vi "range.vi"(9 "2D Pict origin":cluster{"x":dbl, "y":dbl}={"x"=200.0, "y"=200.0}, 10 "L 1":dbl=80.0, 11 "L 2":dbl=80.0) -> (3 "range picture":picture)   [LabVIEW 2024]
panel:
  out "end effector":cluster{dbl, dbl}={159.01647214211073, 1.9100783062530127} {"?" format="%.1f"; "?" format="%#.1f"}
  # "mm"
  # "mm"
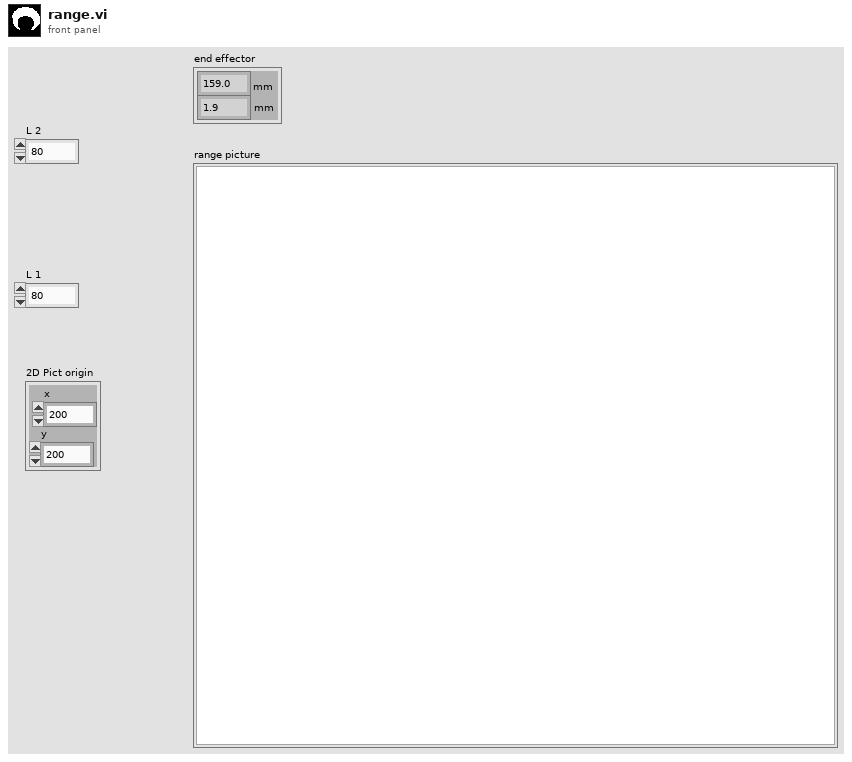
[diagram p1: front panel]
types:
  T1 = cluster{"Width":u16, "Style":enum32{"Solid", "Dash", "Dot", "DashDot", "DashDotDot"}}
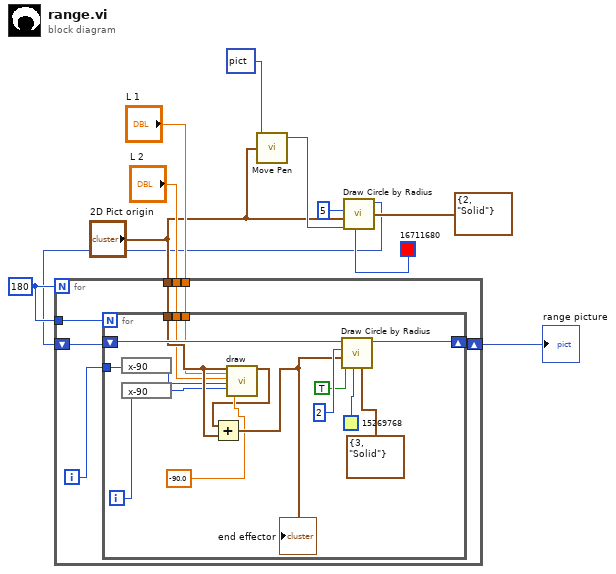
[diagram p0: block diagram]
diagram:
  w7 = 180
  n1 = call <vilib>:"Move Pen.vi"("new position"="2D Pict origin", "picture"=picture data[5B]) -> ("new picture"=w4:picture)  [unwired: 3 in]
  n2 = call <vilib>:"Draw Circle by Radius.vi"("pen"=T1 {"Width"=2, "Style"=enum."Solid"}, "color(black)"=u32 16711680, "pixel center"="2D Pict origin", "radius"=i16 5, "picture"=w4) -> ("new picture"=w1:picture)  [unwired: 6 in]
  n3 = for {
    N: w7 -> [_]
    tunnel: w7 -> [w18]
    shift-right: [w16] -> w6
    shift-left: w1 -> [w17]
    tunnel: "L 1" -> [w14]
    tunnel: "L 2" -> [w13]
    tunnel: "2D Pict origin" -> [w12]
    i -> [w15]
    n4 = for {
      N: w18 -> [_]
      shift-right: [w27] -> w16
      shift-left: w17 -> [w32]
      tunnel: w15 -> [w33]
      tunnel: w14 -> [w24]
      tunnel: w13 -> [w23]
      tunnel: w12 -> [w25]
      i -> [w34]
      n5 = expression code="x-90"(w33) -> (w22:i32)
      n6 = expression code="x-90"(w34) -> (w21:i32)
      n7 = call "draw.vi"("new position"=w25, "L 1"=w24, "L 2"=w23, "Angle1"=w22, "Angle 2"=w21, "bias"=-90.0) -> ("end effector"=w19:cluster{dbl, dbl})  [unwired: 9 in, 4 out]
      n8 = Add(x=w19, y=w25) -> (x+y=w26:cluster{dbl, dbl})
      "end effector" <- w26
      n9 = call <vilib>:"Draw Circle by Radius.vi"("pen"=T1 {"Width"=3, "Style"=enum."Solid"}, "color(black)"=u32 15269768, "fill?(F)"=TRUE, "pixel center"=w26, "radius"=i16 2, "picture"=w32) -> ("new picture"=w27:picture)  [unwired: 5 in]
    }
  }
  "range picture" <- w6
